vi "信号定位.vi"() -> ()   [LabVIEW 2013]
panel:
  out "y":dbl
  out "x":dbl
  in  "y3":dbl
  in  "x3":dbl
  in  "y2":dbl
  in  "x2":dbl
  in  "y1":dbl
  in  "x1":dbl
  in  "signal 3":dbl
  in  "signal 2":dbl
  in  "signal 1":dbl
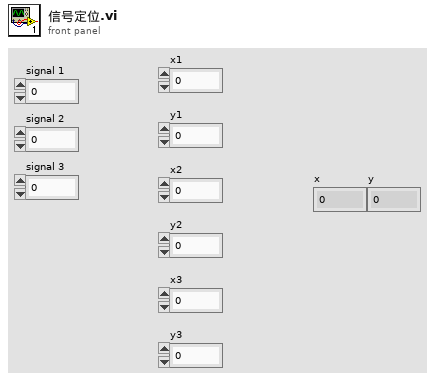
[diagram p1: front panel]
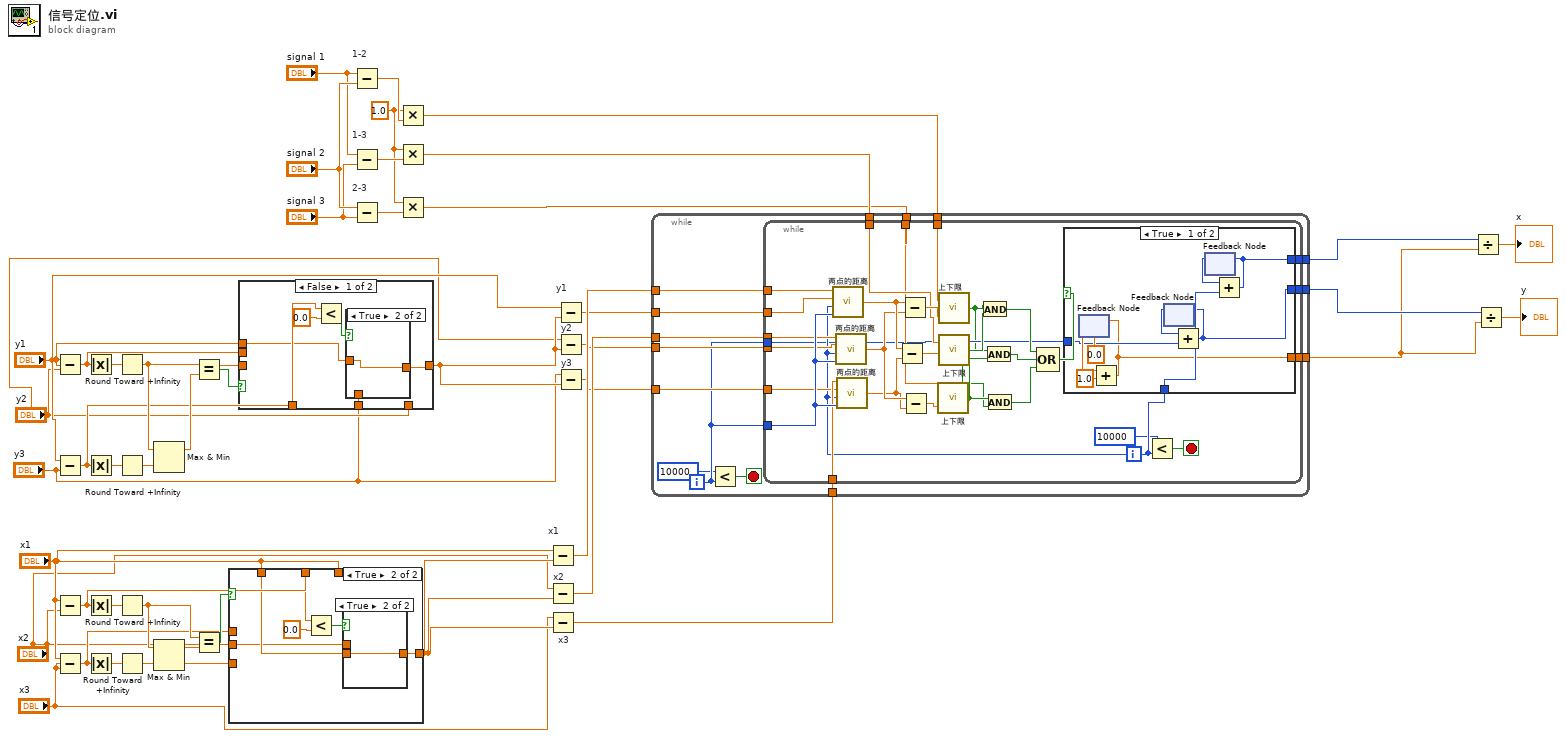
[diagram p0: block diagram]
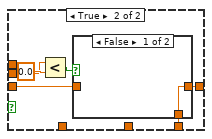
[diagram p3: hidden frame]
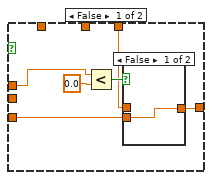
[diagram p5: hidden frame]
diagram:
  w37 = 1.0 ("速度")
  n1 = Subtract(x="y1", y="y2") -> (x-y=w26:dbl)
  n2 = Subtract(x="y1", y="y3") -> (x-y=w25:dbl)
  n3 = Subtract(x="x1", y="x2") -> (x-y=w24:dbl)
  n4 = Subtract(x="x1", y="x3") -> (x-y=w23:dbl)
  n5 = Absolute Value(x=w26) -> (abs(x)=w28:dbl)
  n6 = Absolute Value(x=w25) -> (abs(x)=w27:dbl)
  n7 = Absolute Value(x=w24) -> (abs(x)=w36:dbl)
  n8 = Absolute Value(x=w23) -> (abs(x)=w35:dbl)
  n9 = Round Toward +Infinity(x=w28) -> (ceil(x): smallest int >= x=w29:dbl)
  n10 = Round Toward +Infinity(x=w27) -> (ceil(x): smallest int >= x=w41:dbl)
  n11 = Round Toward +Infinity(x=w36) -> (ceil(x): smallest int >= x=w32:dbl)
  n12 = Round Toward +Infinity(x=w35) -> (ceil(x): smallest int >= x=w42:dbl)
  n13 = Max & Min(x=w29, y=w41) -> (max(x,y)=w30:dbl)  [unwired: 1 out]
  n14 = Max & Min(x=w32, y=w42) -> (max(x,y)=w33:dbl)  [unwired: 1 out]
  n15 = Equal?(x=w29, y=w30) -> (x = y?=w31:bool)
  n16 = Equal?(x=w32, y=w33) -> (x = y?=w34:bool)
  n17 = case shown="True" w34 {
    tunnel: w24 -> [_ w57]
    tunnel: "x1" -> [_ w56]
    tunnel: [w47 w55] -> w22
    tunnel: "x2" -> [_ w54]
    tunnel: w23 -> [w49 _]
    tunnel: "x1" -> [w48 _]
    tunnel: "x3" -> [w46 _]
    frame False {
      n18 = Less?(x=w49, y=0.0) -> (x < y?=w50:bool)
      n19 = case shown="False" w50 {
        tunnel: w48 -> [_ w53]
        tunnel: [w52 w53] -> w47
        tunnel: w46 -> [w52 _]
        frame False {
        }
        frame True {
        }
      }
    }
    frame True {
      n20 = Less?(x=w57, y=0.0) -> (x < y?=w59:bool)
      n21 = case shown="True" w59 {
        tunnel: w56 -> [_ w61]
        tunnel: [w60 w61] -> w55
        tunnel: w54 -> [w60 _]
        frame False {
        }
        frame True {
        }
      }
    }
  }
  n22 = case shown="False" w31 {
    tunnel: w26 -> [_ w73]
    tunnel: "y1" -> [_ w72]
    tunnel: [w63 w71] -> w18
    tunnel: "y2" -> [_ w70]
    tunnel: w25 -> [w65 _]
    tunnel: "y1" -> [w64 _]
    tunnel: "y3" -> [w62 _]
    frame False {
      n23 = Less?(x=w65, y=0.0) -> (x < y?=w66:bool)
      n24 = case shown="True" w66 {
        tunnel: w64 -> [_ w69]
        tunnel: [w68 w69] -> w63
        tunnel: w62 -> [w68 _]
        frame False {
        }
        frame True {
        }
      }
    }
    frame True {
      n25 = Less?(x=w73, y=0.0) -> (x < y?=w75:bool)
      n26 = case shown="False" w75 {
        tunnel: w72 -> [_ w77]
        tunnel: [w76 w77] -> w71
        tunnel: w70 -> [w76 _]
        frame False {
        }
        frame True {
        }
      }
    }
  }
  n27 = Subtract "1-2"(x="signal 1", y="signal 2") -> (x-y=w40:dbl)
  n28 = Subtract "1-3"(x="signal 1", y="signal 3") -> (x-y=w39:dbl)
  n29 = Subtract "2-3"(x="signal 2", y="signal 3") -> (x-y=w38:dbl)
  n30 = Multiply(x=w37, y=w40) -> (x*y=w8:dbl)
  n31 = Multiply(x=w37, y=w39) -> (x*y=w7:dbl)
  n32 = Multiply(x=w37, y=w38) -> (x*y=w6:dbl)
  n33 = Subtract "x1"(x="x1", y=w22) -> (x-y=w14:dbl)
  n34 = Subtract "x2"(x="x2", y=w22) -> (x-y=w12:dbl)
  n35 = Subtract "x3"(x="x3", y=w22) -> (x-y=w10:dbl)
  n36 = Subtract "y1"(x="y1", y=w18) -> (x-y=w13:dbl)
  n37 = Subtract "y2"(x="y2", y=w18) -> (x-y=w11:dbl)
  n38 = Subtract "y3"(x="y3", y=w18) -> (x-y=w9:dbl)
  n39 = while {
    tunnel: w14 -> [w91]
    tunnel: w13 -> [w90]
    tunnel: w12 -> [w89]
    tunnel: w11 -> [w88]
    tunnel: w10 -> [w87]
    tunnel: w9 -> [w86]
    tunnel: w8 -> [w85]
    tunnel: w7 -> [w84]
    tunnel: w6 -> [w83]
    tunnel: [w81] -> w3
    tunnel: [w80] -> w2
    tunnel: [w78] -> w1
    i -> [w82]
    stop <- w92 stop-if-true
    n40 = Less?(x=10000, y=w82) -> (x < y?=w92:bool)
    n41 = while {
      tunnel: w82 -> [w121]
      tunnel: w91 -> [w120]
      tunnel: w90 -> [w119]
      tunnel: w89 -> [w118]
      tunnel: w88 -> [w117]
      tunnel: w87 -> [w116]
      tunnel: w86 -> [w115]
      tunnel: w85 -> [w111]
      tunnel: w84 -> [w108]
      tunnel: w83 -> [w106]
      tunnel: w82 -> [w99]
      tunnel: [w98] -> w81
      tunnel: [w97] -> w80
      tunnel: [w93] -> w78
      i -> [w100]
      stop <- w122 stop-if-true
      n42 = call "两点的距离.vi"("y2"=w121, "x2"=w100, "y1"=w119, "x1"=w120) -> ("de"=w114:dbl)
      n43 = call "两点的距离.vi"("y2"=w121, "x2"=w100, "y1"=w117, "x1"=w118) -> ("de"=w113:dbl)
      n44 = call "两点的距离.vi"("y2"=w121, "x2"=w100, "y1"=w115, "x1"=w116) -> ("de"=w112:dbl)
      n45 = Subtract(x=w114, y=w112) -> (x-y=w109:dbl)
      n46 = Subtract(x=w114, y=w113) -> (x-y=w110:dbl)
      n47 = Subtract(x=w113, y=w112) -> (x-y=w107:dbl)
      n48 = call "上下限.vi"("要比较的"=w107, "范围的中心"=w106) -> ("T/F"=w105:bool)
      n49 = call "上下限.vi"("要比较的"=w110, "范围的中心"=w111) -> ("T/F"=w94:bool)
      n50 = call "上下限.vi"("要比较的"=w109, "范围的中心"=w108) -> ("T/F"=w104:bool)
      n51 = And(x=w94, y=w104) -> (x .and. y?=w103:bool)
      n52 = And(x=w94, y=w105) -> (x .and. y?=w102:bool)
      n53 = And(x=w105, y=w104) -> (x .and. y?=w101:bool)
      n54 = Compound Arithmetic op=OR(w103, w102, w101) -> (w95:bool)
      n55 = case shown="True" w95 {
        tunnel: w100 -> [w126 _]
        tunnel: w99 -> [w129 _]
        tunnel: [w125 _] -> w98
        tunnel: [w124 _] -> w97
        tunnel: [w123 _] -> w93
        frame True {
          n56 = feedback #1(0.0) -> (w132:dbl)
          n57 = Add(x=w132, y=1.0) -> (x+y=w123:dbl)
          n58 = feedback-in #1(w123) -> ()
          n59 = feedback #2() -> (w128:i32)  [unwired: 1 in]
          n60 = Add(x=w128, y=w129) -> (x+y=w124:i32)
          n61 = feedback-in #2(w124) -> ()
          n62 = feedback #3() -> (w127:i32)  [unwired: 1 in]
          n63 = Add(x=w127, y=w126) -> (x+y=w125:i32)
          n64 = feedback-in #3(w125) -> ()
        }
        frame False {
        }
      }
      n65 = Less?(x=10000, y=w100) -> (x < y?=w122:bool)
    }
  }
  n66 = Divide(x=w3, y=w1) -> (x/y=→"x":dbl)
  n67 = Divide(x=w2, y=w1) -> (x/y=→"y":dbl)
